vi "Balance.vi"() -> ()   [LabVIEW 2019]
uses:
  F710PackedLibrary.lvlibp/F710.ctl
  F710PackedLibrary.lvlibp/stick.ctl
  <vilib>/Platform/TimedLoop/XDataNode/timing_clust.ctl
  <vilib>/Platform/TimedLoop/XDataNode/nitl_modes.ctl
  <vilib>/Platform/TimedLoop/XDataNode/wakeup.ctl
  F710PackedLibrary.lvlibp/gamepadF710.lvclass
  KNRm_ReMi_OS6_436Motor.lvlibp/KNRm_ReMi_Toolkit/IO/LowLevel/IO_Channel_DIO.ctl
  KNRm_ReMi_OS6_436Motor.lvlibp/KNRm_ReMi_Toolkit/IO/LowLevel/IOSETChannel.ctl
  KNRm_ReMi_OS6_436Motor.lvlibp/KNRm_ReMi_Toolkit/IO/LowLevel/IO_Channel_RC.ctl
  <vilib>/Analysis/3filter.llb/Filter Passband Type.ctl
  <vilib>/addons/control/pid/pid.llb/PID (DBL).vi
  <vilib>/platform/TimedLoop/XDataNode/XDataNode.xnode
  <vilib>/Platform/TimedLoop/XDataNode/XDNodeRunTimeDep.lvlib
  KNRm_ReMi_OS6_436Motor.lvlibp/BNO055_KNRm_ReMi.lvlib
  KNRm_ReMi_OS6_436Motor.lvlibp
  <vilib>/ptbypt/NI_PtbyPt.lvlib
  <vilib>/Analysis/NI_AALBase.lvlib
  <vilib>/addons/control/pid/NI_PID_pid.lvlib
  F710PackedLibrary.lvlibp
panel:
  out "Gyro":dbl=9.0
  in  "Degreecontrol":T1={"proportional gain (Kc)"=180.0, "integral time (Ti, min)"=0.00121, "derivative time (Td, min)"=0.0}
  in  "Speedcontrol":T1={"proportional gain (Kc)"=0.102, "integral time (Ti, min)"=0.002, "derivative time (Td, min)"=0.0}
  in  "GyroOffset":dbl=9.0
  out "MotorSpeed":dbl=-7.875
  out "Axis info.Right x-Axis":i8
  out "tel":dbl=9.0
  out "ªûÁ³»öÂoªi":cluster{dbl, "Filtered x":dbl}(graph)={1.1875, "Filtered x"=1.3918305965663234}
  out "F710 button info.left":bool
  out "F710 button info.right":bool
  out "F710 button info.B":bool
  out "F710 button info.X":bool
  out "F710 button info.Y":bool
  out "F710 button info.down":bool
  out "F710 button info.up":bool
  out "RT-LT":dbl
  out "Axis info.Left y-Axis":i8
  out "F710 button info.back":bool
  out "F710 button info.start":bool
  out "error out":errorcluster
  out "F710":T2
  out "Control Late?":bool=TRUE
  # "¦³µo®g           ¨Sµo®g"
  # "180               160\n\n0.00121   0.00125\n\n0                      0\n\n\n\n\n\n0.102           0.034\n \n0.002            0.01\n\n0                      0"
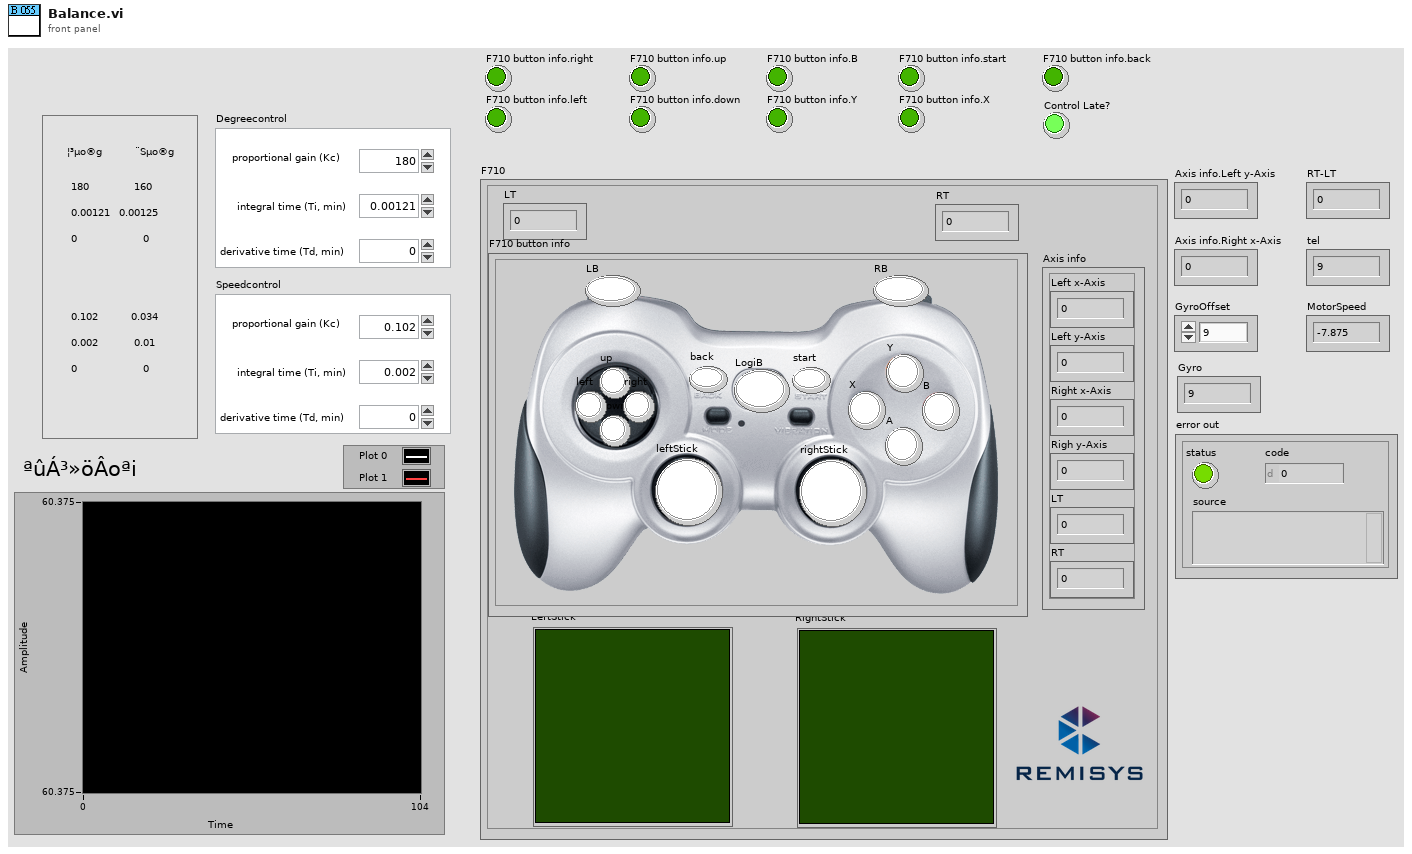
[diagram p1: front panel]
types:
  T1 = cluster{"proportional gain (Kc)":dbl, "integral time (Ti, min)":dbl, "derivative time (Td, min)":dbl}
  T2 = typedef "F710PackedLibrary.lvlibp/F710.ctl" = cluster{"RT":u8, "LT":u8, "RightStick":T3, "LeftStick":T3, "Axis info":cluster{"Left x-Axis":i8, "Left y-Axis":i8, "Right x-Axis":i8, "Righ y-Axis":i8, "LT":u8, "RT":u8}, "F710 button info":cluster{"RB":bool, "LB":bool, "rightStick":bool, "leftStick":bool, "start":bool, "back":bool, "right":bool, "left":bool, "down":bool, "up":bool, "Y":bool, "X":bool, "B":bool, "A":bool, "LogiB":bool}}
  T3 = typedef "F710PackedLibrary.lvlibp/stick.ctl" = cluster{"X":dbl, "Y":dbl}[]
  T4 = typedef "KNRm_ReMi_OS6_436Motor.lvlibp/IO_Channel_RC.ctl" = enum16{"RC1", "RC2", "S1(EXTIOB)", "S2(EXTIOB)", "S3(EXTIOB)", "S4(EXTIOB)", "S5(EXTIOB)", "S6(EXTIOB)"}
  T5 = typedef "KNRm_ReMi_OS6_436Motor.lvlibp/IOSETChannel.ctl" = enum8{"0:B_DIO1/M1.EN/SM6.PULSE.CH1", "1:A_DIO8/M2.EN/SM6.DIR.CH1", "2:B_DIO7/M3.EN/SM6.PULSE.CH2", "3:A_DIO3/M4.EN/SM6.DIR.CH2", "4:A_DIO14/RC1_0", "5:A_DIO15/RC1_1", "6:LED(4)"}
  T6 = cluster{T5, "Checkbox":bool, "CycleTick":fxp<+,22,22>, "DutyCycleTick":fxp<+,22,22>}[]
  T7 = typedef "KNRm_ReMi_OS6_436Motor.lvlibp/IO_Channel_DIO.ctl" = enum16{"B/DIO1 (M1)", "A/DIO8 (M2)", "B/DIO7 (M3)", "A/DIO3 (M4)", "A/DIO14 (RC1_0)", "A/DIO15 (RC1_1)", "A/DIO7(S1)", "A/DIO2(S2)", "A/DIO6(S3)", "A/DIO3(S4)", "A/DIO5(S5)", "A/DIO4(S6)"}
  T8 = enum16{"ConfigMode", "ACC only", "Mag only", "Gyro only", "Acc Mag", "Acc Gyro", "Mag Gyro", "AMG", "Fusion IMU", "Fusion Compass", "Fusion M4G", "NDOF_FMC_OFF", "NDOF"}
  T9 = typedef "XDNodeRunTimeDep.lvlib/timing_clust.ctl" = cluster{"Expected End [f-1]":u64, "Actual End [f-1]":u64, "Finished Late? [f-1]":bool, "Expected End [i-1]":u64, "Actual End [i-1]":u64, "Finished Late? [i-1]":bool, "Expected Start [i]":u64, "Actual Start [i]":u64, "Expected Start [f]":u64, "Actual Start [f]":u64, "Source Name":string, "Structure Name":string, "Period":i64, "Deadline":i64, "Offset":i64, "Start":i64, "Priority":i32, "Timeout":i32, "Mode":T10, "Wakeup Reason":T11, "Error":errorcluster, "Source Type":string, "Secondary Source Type":string, "Global End Time":u64, "Global Start Time":u64, "Frame Duration":u64, "Iteration Duration":u64, "Assigned CPU":i32, "I/O Scan Engine Mode":u32}
  T10 = typedef "XDNodeRunTimeDep.lvlib/nitl_modes.ctl" = enum32{"No Change", "Process missed periods, maintain original phase", "Discard missed periods, maintain original phase", "Process missed periods, ignore original phase", "Discard missed periods, ignore original phase"}
  T11 = typedef "XDNodeRunTimeDep.lvlib/wakeup.ctl" = enum32{"Normal", "Aborted", "Asynchronous wakeup", "Timing source error", "Timed loop error", "Timeout"}
  T12 = cluster{T5, "Checkbox":bool, "CycleTick":fxp<+,22,22>, "DutyCycleTick":fxp<+,22,22>}
  T13 = cluster{T5, "Checkbox":bool, "CycleTick":fxp<+,22,22>, "f":fxp<+,22,22>}
  T14 = cluster{T5, "Checkbox":bool, "CycleTick":fxp<+,22,22>, "f":fxp<+,22,22>}[]
  T15 = typedef "NI_AALBase.lvlib/Filter Passband Type.ctl" = enum32{"Lowpass", "Highpass", "Bandpass", "Bandstop"}
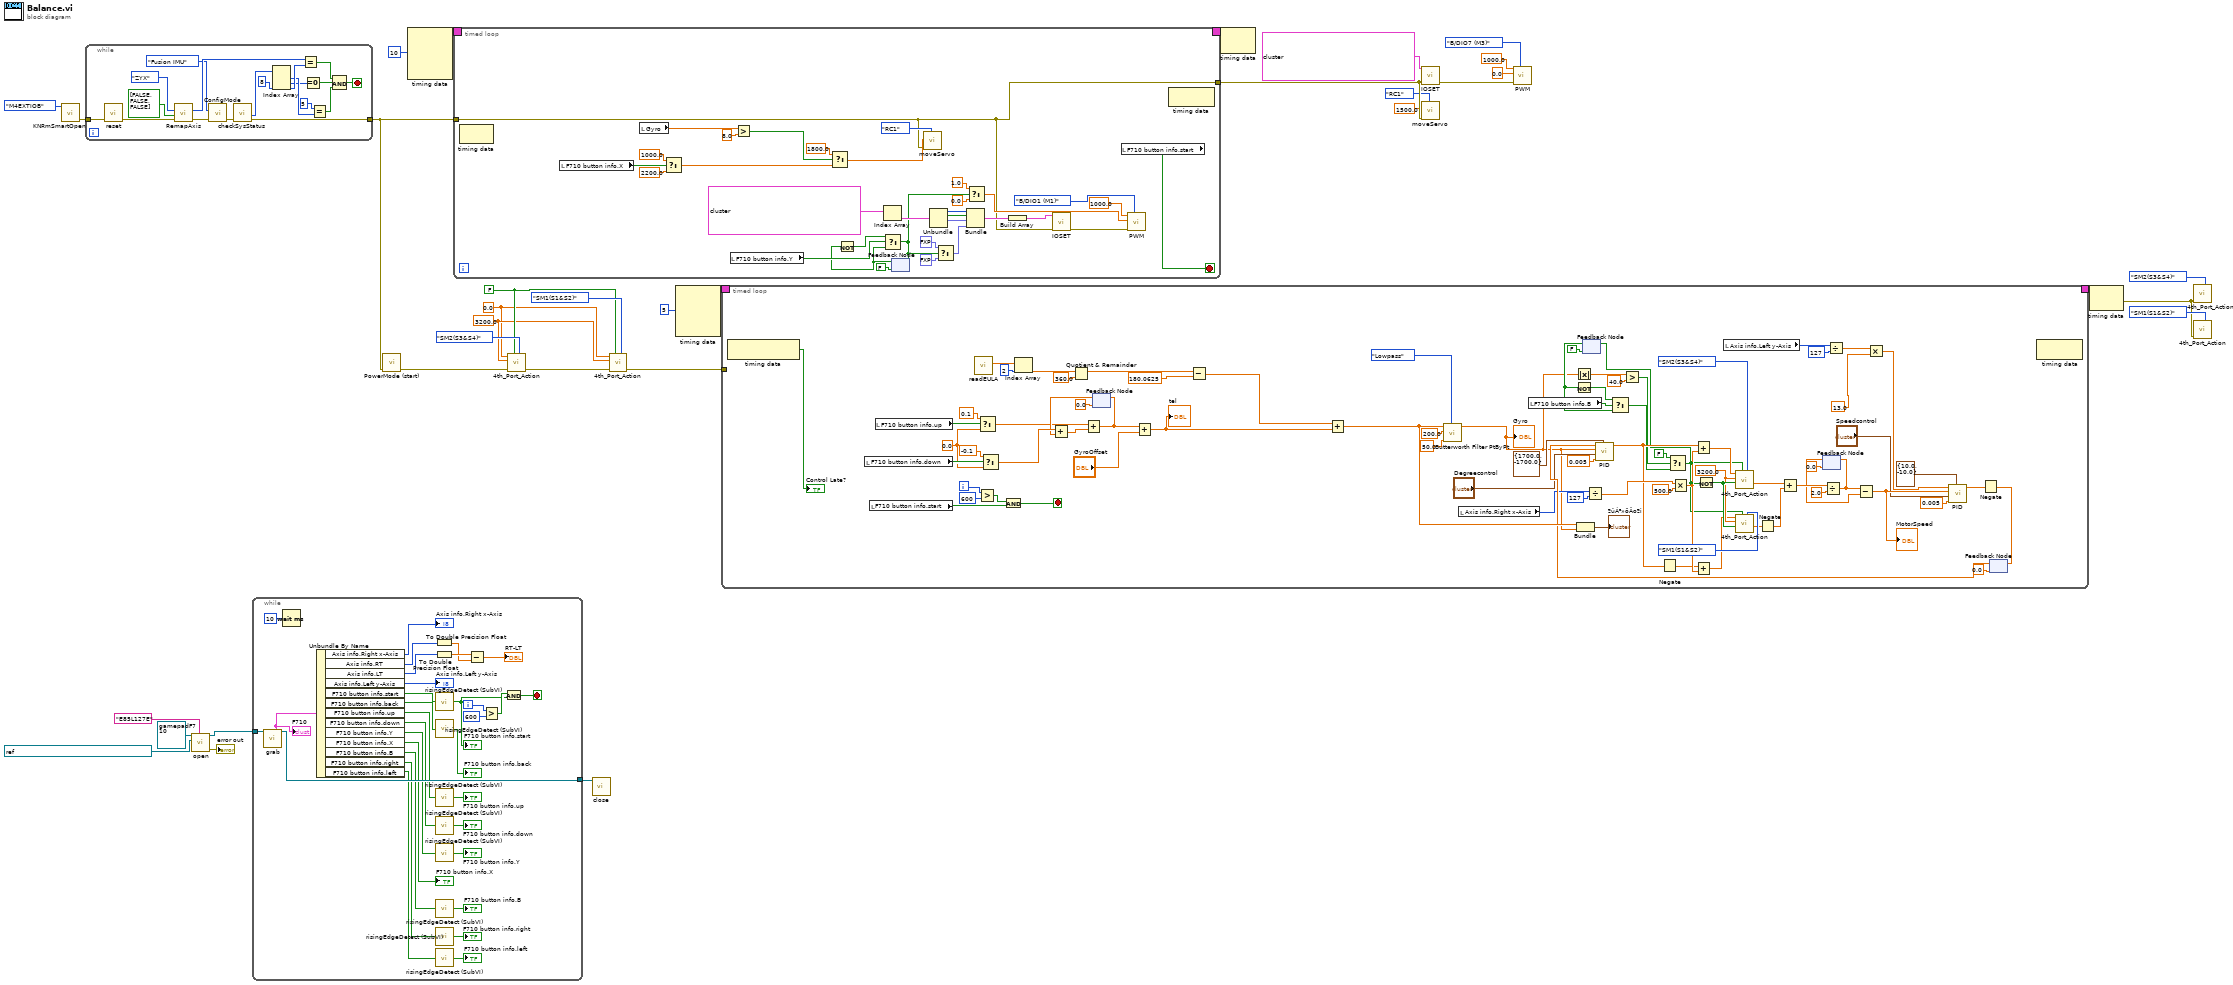
[diagram p0: block diagram]
diagram:
  w7 = 0.0 ("vel(deg/sec)")
  w8 = 3200.0 ("vel(deg/sec)")
  w9 = FALSE ("EN")
  n1 = call "KNRmSmartOpen.vi"("INI FPGA MODE"=enum16{"Original", "M4EXTIOB"}."M4EXTIOB") -> ("error out"=w16:errorcluster)  [unwired: 7 in, 3 out]
  n2 = while {
    tunnel: [w36] -> w6
    tunnel: w16 -> [w35]
    stop <- w52 stop-if-true
    n3 = call "reset.vi"("error in (no error)"=w35) -> ("error out"=w42:errorcluster)  [unwired: 10 in]
    n4 = call "RemapAxis.vi"("error in (no error)"=w42, "AxisSign [X, Y, Z] ( F:Pos, T:Neg)"=bool[] [FALSE, FALSE, FALSE], "AxisRemap [ Z, Y, X]"=enum16{"XYZ", "XZY", "YXZ", "YZX", "ZXY", "ZYX"}."ZYX" ("AxisRemap")) -> ("Error Out"=w39:errorcluster, "hexOut"=w41:u8)  [unwired: 7 in]
    n5 = call "ConfigMode.vi"("error in (no error)"=w39, "Mode"=T8."Fusion IMU") -> ("error out"=w38:errorcluster)  [unwired: 9 in]
    n6 = call "checkSysStatus.vi"("error in (no error)"=w38) -> ("error out"=w36:errorcluster, "System Status code"=w37:u8[])  [unwired: 8 in, 1 out]
    n7 = Index Array(array=w37, index #3=8 ("index")) -> (element #1=w49:u8, element #2=w47:u8, element #3=w50:u8)  [unwired: 2 in]
    n8 = Equal?(x=w41, y=w50) -> (x = y?=w53:bool)
    n9 = Equal To 0?(x=w47) -> (x = 0?=w46:bool)
    n10 = Equal?(x=u8 5, y=w49) -> (x = y?=w45:bool)
    n11 = Compound Arithmetic op=AND(w53, w46, w45) -> (w52:bool)
  }
  n12 = call "open.vi"("INPUT S/N"="E85L127E", "VISA resource name"=refnum<visa-resource-name> "USB0::0x046D::0xC21F::9BD89EBC::RAW", "gamepadF710 in"=refnum<class "gamepadF710.lvclass"> refnum) -> ("error out"=→"error out":errorcluster, "gamepadF710 out"=w27:refnum<class "gamepadF710.lvclass">)  [unwired: 6 in, 1 out]
  n13 = while {
    tunnel: w27 -> [w85]
    tunnel: [w84] -> w26
    i -> [w80]
    stop <- w78 stop-if-true
    n14 = call "grab.vi"("gamepadF710 in"=w85) -> ("gamepadF710 out"=w84:refnum<class "gamepadF710.lvclass">, "F710"=w82:T2)  [unwired: 7 in, 1 out]
    "F710" <- w82
    n15 = Wait (ms)(milliseconds to wait=u32 10) -> ()  [unwired: 1 out]
    n16 = Unbundle By Name(w82) -> ("Axis info.Right x-Axis"=→"Axis info.Right x-Axis":i8, "Axis info.RT"=w76:u8, "Axis info.LT"=w75:u8, "Axis info.Left y-Axis"=→"Axis info.Left y-Axis":i8, "F710 button info.start"=w63:bool, "F710 button info.back"=w62:bool, "F710 button info.up"=w67:bool, "F710 button info.down"=w65:bool, "F710 button info.Y"=w69:bool, "F710 button info.X"=→"F710 button info.X":bool, "F710 button info.B"=w55:bool, "F710 button info.right"=w70:bool, "F710 button info.left"=w71:bool)
    n17 = To Double Precision Float(number=w76) -> (double precision float=w57:dbl)
    n18 = To Double Precision Float(number=w75) -> (double precision float=w58:dbl)
    n19 = call "risingEdgeDetect (SubVI).vi"("input"=w63) -> ("output"=w60:bool)
    "F710 button info.start" <- w60
    n20 = call "risingEdgeDetect (SubVI).vi"("input"=w62) -> ("output"=→"F710 button info.back":bool)
    n21 = call "risingEdgeDetect (SubVI).vi"("input"=w67) -> ("output"=→"F710 button info.up":bool)
    n22 = call "risingEdgeDetect (SubVI).vi"("input"=w65) -> ("output"=→"F710 button info.down":bool)
    n23 = call "risingEdgeDetect (SubVI).vi"("input"=w69) -> ("output"=→"F710 button info.Y":bool)
    n24 = call "risingEdgeDetect (SubVI).vi"("input"=w55) -> ("output"=→"F710 button info.B":bool)
    n25 = call "risingEdgeDetect (SubVI).vi"("input"=w70) -> ("output"=→"F710 button info.right":bool)
    n26 = call "risingEdgeDetect (SubVI).vi"("input"=w71) -> ("output"=→"F710 button info.left":bool)
    n27 = Subtract(x=w58, y=w57) -> (x-y=→"RT-LT":dbl)
    n28 = Greater?(x=w80, y=600) -> (0:w77:bool)
    n29 = And(x=w77, y=w60) -> (x .and. y?=w78:bool)
  }
  n30 = call "PowerMode (start).vi"("error in (no error)"=w6) -> ("error out"=w14:errorcluster)  [unwired: 10 in]
  n31 = node-c288(i64 10 ("Period")) -> (w25:T9)  [unwired: 3 in]
  n32 = timed-loop {
    timing: w25 -> [_]
    timing-out: [_] -> w24
    tunnel: w6 -> [w87]
    tunnel: [w87] -> w3
    stop <- w118 stop-if-true
    n33 = node-c288() -> ()  [unwired: 1 in, 1 out]
    n34 = local read "F710 button info.X"() -> (w117:bool)
    n35 = local read "Gyro"() -> (w89:dbl)
    n36 = Select(t=1000.0, s=w117, f=2200.0) -> (s? t:f=w93:dbl)
    n37 = local read "F710 button info.Y"() -> (w106:bool)
    n38 = Greater?(x=w89, y=8.0) -> (0:w90:bool)
    n39 = Select(t=1800.0, s=w90, f=w93) -> (s? t:f=w92:dbl)
    n40 = Index Array(array=T6 [{enum."0:B_DIO1/M1.EN/SM6.PULSE.CH1", "Checkbox"=TRUE, "CycleTick"=0.0, "DutyCycleTick"=0.0}] ("IOSET")) -> (element=w112:T12)  [unwired: 1 in]
    n41 = feedback #1(FALSE ("F710 button info.Y")) -> (w103:bool)
    n42 = Not(x=w103) -> (.not. x?=w104:bool)
    n43 = Select(t=w104, s=w106, f=w103) -> (s? t:f=w97:bool)
    n44 = feedback-in #1(w97) -> ()
    n45 = call "moveServo.vi"("Channel"=IO_Channel_RC."RC1", "error in (no error)"=w87, "Servo Position (us)"=w92) -> ()  [unwired: 8 in, 1 out]
    n46 = Unbundle(w112) -> (w111:T5, "Checkbox"=w110:bool, "CycleTick"=w109:fxp<+,22,22>)  [unwired: 1 out]
    n47 = Select(t=fxp<+,22,22> 1.0, s=w97, f=fxp<+,22,22> 0.0) -> (s? t:f=w100:fxp<+,22,22>)
    n48 = Bundle(w111, "Checkbox"=w110, "CycleTick"=w109, "f"=w100) -> (w108:T13)  [unwired: 1 in]
    n49 = Select(t=1.0 ("DutyCycle"), s=w97, f=0.0 ("DutyCycle")) -> (s? t:f=w94:dbl)
    n50 = Build Array(w108) -> (w107:T14)
    n51 = call "IOSET.vi"("error in"=w87, "IOSET"=w107) -> ("error out"=w86:errorcluster)  [unwired: 8 in, 1 out]
    n52 = local read "F710 button info.start"() -> (w118:bool)
    n53 = call "PWM.vi"("IO_Chanel"=IO_Channel_DIO."B/DIO1 (M1)", "error in"=w86, "DutyCycle"=w94, "Frequency(Hz)"=1000.0) -> ()  [unwired: 7 in, 1 out]
    n54 = node-c288() -> ()  [unwired: 1 in, 1 out]
  }
  n55 = call "4th_Port_Action.vi"("Port"=enum16{"SM1(S1&S2)", "SM2(S3&S4)", "SM3(S5&S6)"}."SM2(S3&S4)", "EN"=w9, "error in"=w14, "step"=w8, "vel(deg/sec)"=w7) -> ("error out"=w13:errorcluster)  [unwired: 4 in, 2 out]
  n56 = call "close.vi"("gamepadF710 in"=w26) -> ()  [unwired: 9 in, 2 out]
  n57 = call "4th_Port_Action.vi"("Port"=enum16{"SM1(S1&S2)", "SM2(S3&S4)", "SM3(S5&S6)"}."SM1(S1&S2)", "EN"=w9, "error in"=w13, "step"=w8, "vel(deg/sec)"=w7) -> ("error out"=w12:errorcluster)  [unwired: 4 in, 2 out]
  n58 = node-c288(i64 5 ("Period")) -> (w34:T9)  [unwired: 3 in]
  n59 = timed-loop {
    timing: w34 -> [_]
    timing-out: [_] -> w33
    tunnel: w12 -> [_]
    i -> [w198]
    stop <- w138 stop-if-true
    w146 = 3200.0 ("step")
    w174 = 0.0 ("offset")
    n60 = node-c288() -> (→"Control Late?":bool)  [unwired: 1 in]
    n61 = local read "F710 button info.down"() -> (w180:bool)
    n62 = local read "F710 button info.start"() -> (w189:bool)
    n63 = local read "F710 button info.up"() -> (w182:bool)
    n64 = call "readEULA.vi"() -> ("EULA Output"=w192:dbl[])  [unwired: 10 in, 1 out]
    n65 = Select(t=0.1, s=w182, f=w174) -> (s? t:f=w175:dbl)
    n66 = Greater?(x=w198, y=600) -> (0:w196:bool)
    n67 = Select(t=-0.1, s=w180, f=w174) -> (s? t:f=w178:dbl)
    n68 = And(x=w196, y=w189) -> (x .and. y?=w138:bool)
    n69 = Index Array(array=w192, index=2) -> (element=w193:dbl)
    n70 = Quotient & Remainder(x=w193, y=360.0) -> (x-y*floor(x/y)=w188:dbl)  [unwired: 1 out]
    n71 = feedback #2(0.0 ("y")) -> (w177:dbl)
    n72 = Add(x=w178, y=w177) -> (x+y=w176:dbl)
    n73 = Add(x=w175, y=w176) -> (x+y=w153:dbl)
    n74 = feedback-in #2(w153) -> ()
    n75 = Add(x=w153, y="GyroOffset") -> (x+y=w151:dbl)
    "tel" <- w151
    n76 = Subtract(x=w188, y=180.0625) -> (x-y=w190:dbl)
    n77 = Add(x=w190, y=w151) -> (x+y=w184:dbl)
    n78 = call <vilib>:"Butterworth Filter PtByPt.vi"("filter type"=Filter_Passband_Type."Lowpass", "low cutoff freq: fl"=50.0, "sampling freq: fs"=200.0, "x"=w184) -> ("Filtered x"=w129:dbl)  [unwired: 5 in, 1 out]
    "Gyro" <- w129
    n79 = local read "Axis info.Right x-Axis"() -> (w150:i8)
    n80 = local read "F710 button info.B"() -> (w126:bool)
    n81 = Absolute Value(x=w129) -> (abs(x)=w128:dbl)
    n82 = Bundle(w184, "Filtered x"=w129) -> (→"ªûÁ³»öÂoªi":cluster{dbl, "Filtered x":dbl})  [unwired: 1 in]
    n83 = feedback #3(FALSE ("EnableMotor")) -> (w132:bool)
    n84 = Not(x=w132) -> (.not. x?=w133:bool)
    n85 = Divide(x=w150, y=i8 127) -> (x/y=w148:dbl)
    n86 = Select(t=w133, s=w126, f=w132) -> (s? t:f=w123:bool)
    n87 = Greater?(x=w128, y=40.0) -> (0:w125:bool)
    n88 = Select(t=FALSE ("EnableMotor"), s=w125, f=w123) -> (s? t:f=w122:bool)
    n89 = feedback-in #3(w122) -> ()
    n90 = Multiply(x=w148, y=500.0) -> (x*y=w143:dbl)
    n91 = Not(x=w122) -> (.not. x?=w171:bool)
    n92 = local read "Axis info.Left y-Axis"() -> (w139:i8)
    n93 = feedback #4(0.0) -> (w163:dbl)
    n94 = Divide(x=w139, y=i8 127) -> (x/y=w131:dbl)
    n95 = Multiply(x=w131, y=13.0) -> (x*y=w130:dbl)
    n96 = feedback #5(0.0 ("output")) -> (w157:dbl)
    n97 = call-poly <vilib>:"PID.vi"("output range"=cluster{"output high":dbl, "output low":dbl} {"output high"=1700.0, "output low"=-1700.0}, "dt (s)"=0.005, "PID gains"="Degreecontrol", "process variable"=w129, "setpoint"=w157) -> ("output"=w145:dbl)  [unwired: 5 in, 1 out]
    n98 = Negate(x=w145) -> (-x=w141:dbl)
    n99 = Add(x=w145, y=w143) -> (x+y=w144:dbl)
    n100 = Add(x=w141, y=w143) -> (x+y=w142:dbl)
    n101 = call "4th_Port_Action.vi"("Port"=enum16{"SM1(S1&S2)", "SM2(S3&S4)", "SM3(S5&S6)"}."SM2(S3&S4)", "EN"=w122, "ResetCounter"=w171, "step"=w146, "vel(deg/sec)"=w144) -> ("motordegree"=w169:dbl)  [unwired: 4 in, 2 out]
    n102 = call "4th_Port_Action.vi"("Port"=enum16{"SM1(S1&S2)", "SM2(S3&S4)", "SM3(S5&S6)"}."SM1(S1&S2)", "EN"=w122, "ResetCounter"=w171, "step"=w146, "vel(deg/sec)"=w142) -> ("motordegree"=w170:dbl)  [unwired: 4 in, 2 out]
    n103 = Negate(x=w170) -> (-x=w168:dbl)
    n104 = Add(x=w169, y=w168) -> (x+y=w167:dbl)
    n105 = Divide(x=w167, y=2.0) -> (x/y=w158:dbl)
    n106 = feedback-in #4(w158) -> ()
    n107 = Subtract(x=w158, y=w163) -> (x-y=w159:dbl)
    "MotorSpeed" <- w159
    n108 = call-poly <vilib>:"PID.vi"("output range"=cluster{"output high":dbl, "output low":dbl} {"output high"=10.0, "output low"=-10.0}, "dt (s)"=0.005, "PID gains"="Speedcontrol", "process variable"=w159, "setpoint"=w130) -> ("output"=w156:dbl)  [unwired: 5 in, 1 out]
    n109 = Negate(x=w156) -> (-x=w135:dbl)
    n110 = feedback-in #5(w135) -> ()
    n111 = node-c288() -> ()  [unwired: 1 in, 1 out]
  }
  n112 = node-c288(w24) -> ()  [unwired: 1 out]
  n113 = call "IOSET.vi"("error in"=w3, "IOSET"=T6 [{enum."0:B_DIO1/M1.EN/SM6.PULSE.CH1", "Checkbox"=TRUE, "CycleTick"=0.0, "DutyCycleTick"=0.0}]) -> ("error out"=w5:errorcluster)  [unwired: 8 in, 1 out]
  n114 = call "moveServo.vi"("Channel"=IO_Channel_RC."RC1", "error in (no error)"=w3, "Servo Position (us)"=1500.0) -> ()  [unwired: 8 in, 1 out]
  n115 = call "PWM.vi"("IO_Chanel"=IO_Channel_DIO."B/DIO7 (M3)", "error in"=w5, "DutyCycle"=0.0, "Frequency(Hz)"=1000.0) -> ()  [unwired: 7 in, 1 out]
  n116 = node-c288(w33) -> (w20:errorcluster)
  n117 = call "4th_Port_Action.vi"("Port"=enum16{"SM1(S1&S2)", "SM2(S3&S4)", "SM3(S5&S6)"}."SM2(S3&S4)", "error in"=w20) -> ()  [unwired: 7 in, 3 out]
  n118 = call "4th_Port_Action.vi"("Port"=enum16{"SM1(S1&S2)", "SM2(S3&S4)", "SM3(S5&S6)"}."SM1(S1&S2)", "error in"=w20) -> ()  [unwired: 7 in, 3 out]
